vi "AttrMap-Preview.vi"(8 "error in (no error)":errorcluster, 11 "AttrMap in":T1) -> (0 "error out":errorcluster, 3 "AttrMap out":T1)   [LabVIEW 2019, in "lv-apt-json-file.lvlib"]
uses:
  lv-apt-json-file.lvlib
  Def-AttrMap.ctl
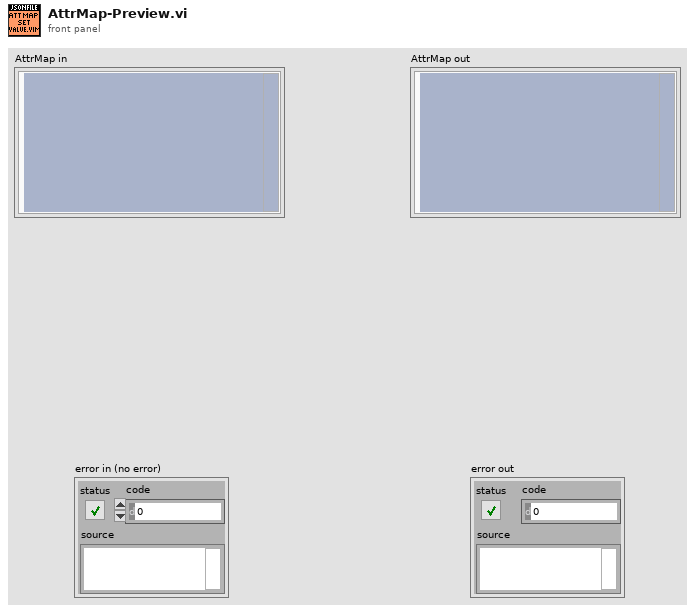
[diagram p1: front panel]
types:
  T1 = typedef "lv-apt-json-file.lvlib/Def-AttrMap.ctl" = cluster{"Map":variant}
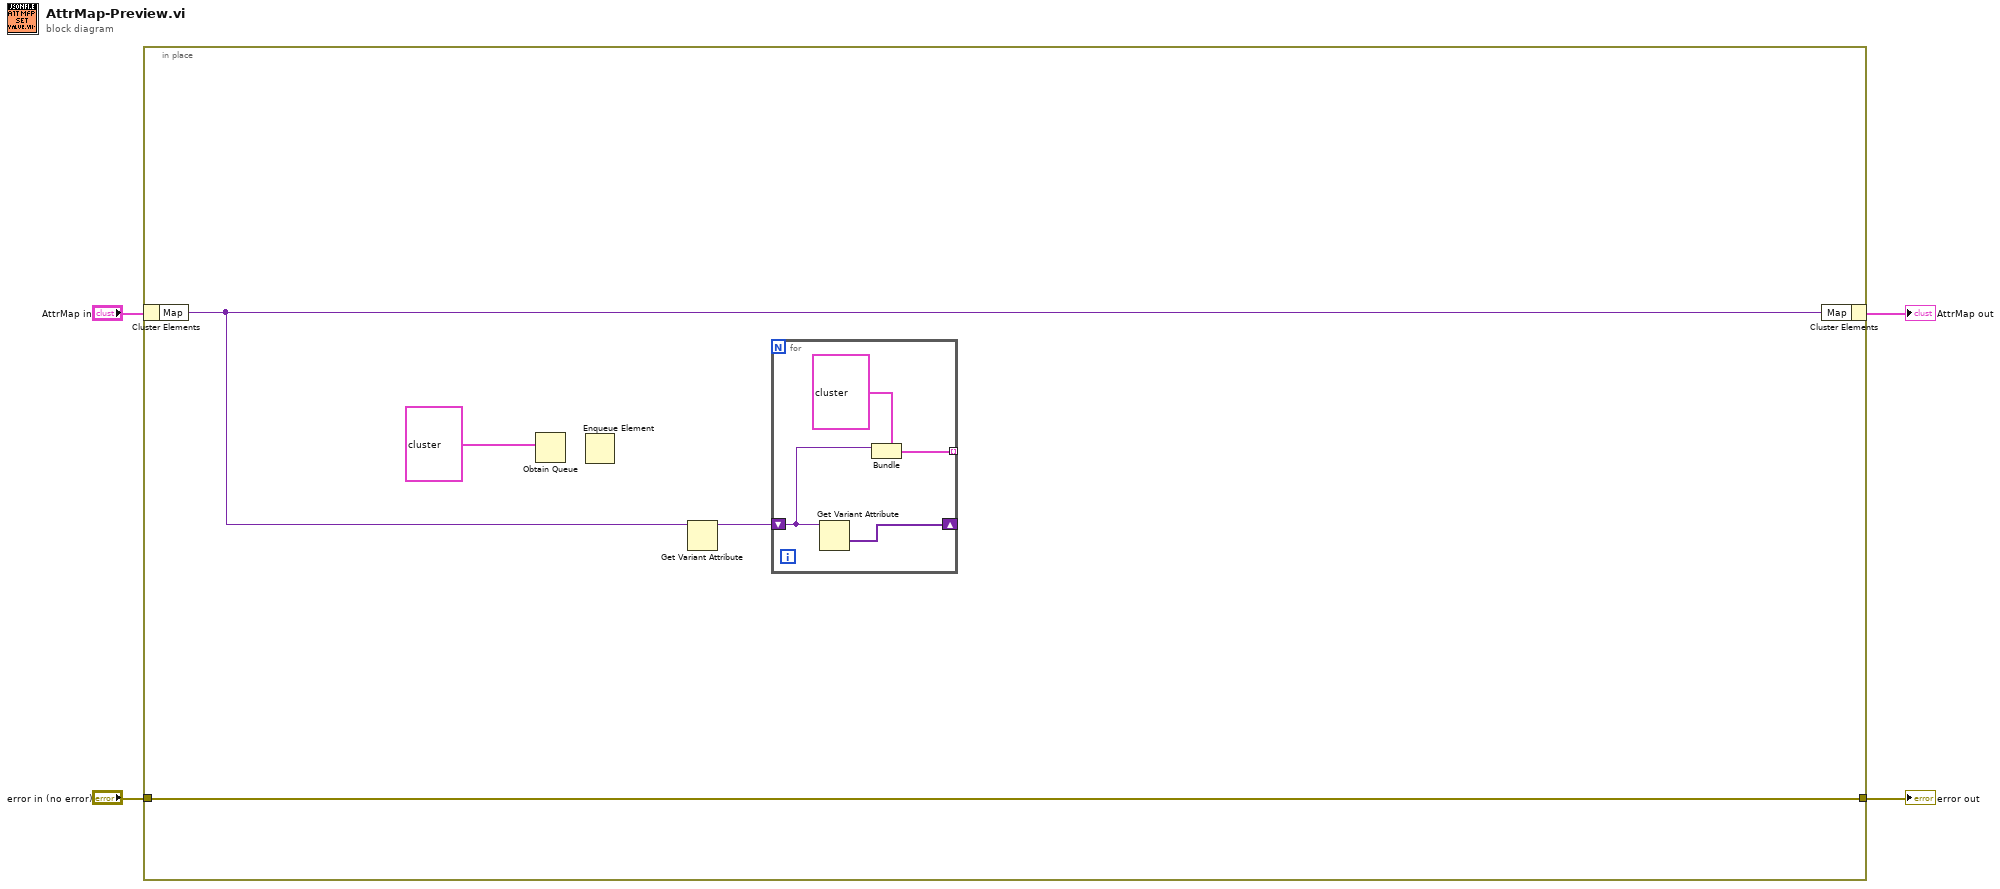
[diagram p0: block diagram]
diagram:
  n1 = in-place {
    in-place-border: [w8] -> w4
    in-place-border: "error in (no error)" -> [w8]
    n2 = in-place-cluster #1("AttrMap in") -> ("Map"=w6:variant)
    n3 = Obtain Queue(element data type=cluster{"Parent":variant, "Name":string} {"Parent"=variant, "Name"=""}) -> ()  [unwired: 4 in, 3 out]
    n4 = Enqueue Element() -> ()  [unwired: 4 in, 3 out]
    n5 = Get Variant Attribute(Variant=w6) -> (duplicate Variant=w5:variant)  [unwired: 3 in, 3 out]
    n6 = for {
      shift-right: [w11] -> _
      shift-left: w5 -> [w12]
      tunnel: [w9] -> _ mode=indexing
      n7 = Get Variant Attribute(Variant=w12) -> (values=w11:variant[])  [unwired: 3 in, 3 out]
      n8 = Bundle(cluster=cluster{"Parent":variant, "Name":string} {"Parent"=variant, "Name"=""}, "Parent"=w12) -> (w9:cluster{"Parent":variant, "Name":string})  [unwired: 1 in]
    }
    n9 = in-place-cluster #1("Map"=w6) -> (→"AttrMap out":T1)
  }
  "error out" <- w4
